vi "FFT(SubVI).vi"(0 "Data in":dbl[](array[numeric]), 1 "Window":u16, 2 "FFT size":i32, 3 "Sampling freq":dbl, 4 "Nyqvist Zone":enum32{"Zone 1", "Zone 2"}(radio)) -> (5 "Freq axis":dbl[](array[numeric]), 6 "FFT":dbl[](array[numeric]), 7 "DC Element":dbl)   [LabVIEW 2013]
uses:
  <vilib>/Analysis/4window.llb/Blackman Window (DBL).vi
  <vilib>/Analysis/4window.llb/Blackman-Harris Window (DBL).vi
  <vilib>/Analysis/4window.llb/Hamming Window (DBL).vi
  <vilib>/Analysis/4window.llb/Hanning Window (DBL).vi
  <vilib>/Analysis/2dsp.llb/Real FFT.vi
  <vilib>/Analysis/4window.llb/AllCosWindow (DBL).vi
  <vilib>/Analysis/NI_AALPro.lvlib
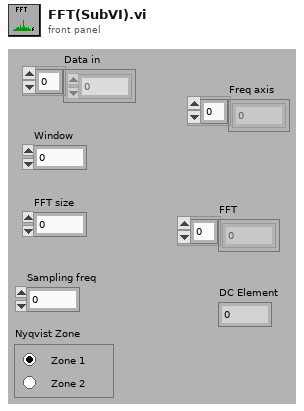
[diagram p1: front panel]
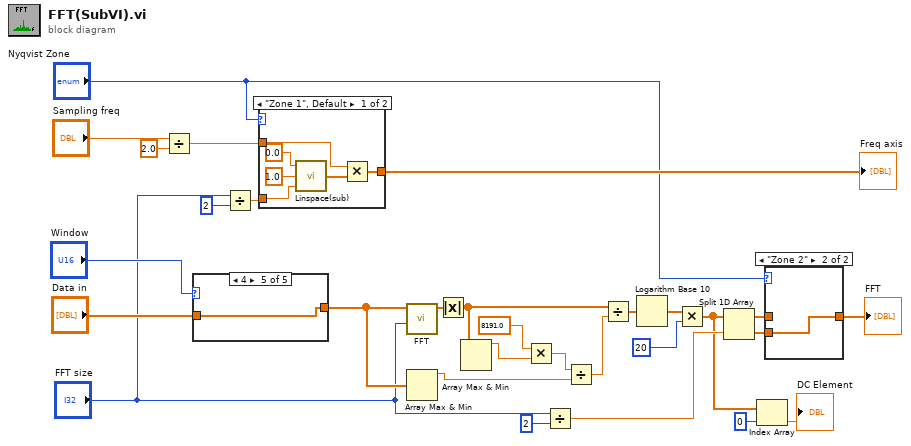
[diagram p0: block diagram]
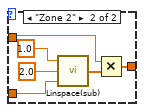
[diagram p3: hidden frame]
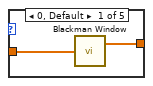
[diagram p4: hidden frame]
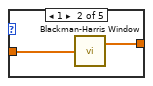
[diagram p5: hidden frame]
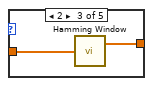
[diagram p6: hidden frame]
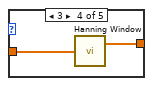
[diagram p7: hidden frame]
diagram:
  n1 = Divide(x="Sampling freq", y=2.0) -> (x/y=w17:dbl)
  n2 = case shown="4" "Window" {
    tunnel: [w31 w33 w35 w37 w38] -> w16
    tunnel: "Data in" -> [w30 w32 w34 w36 w38]
    frame 0, Default {
      n3 = call-poly <vilib>:"Blackman Window.vi"("X"=w30) -> ("Windowed X"=w31:dbl[])  [unwired: 1 out]
    }
    frame 1 {
      n4 = call-poly <vilib>:"Blackman-Harris Window.vi"("X"=w32) -> ("Windowed X"=w33:dbl[])  [unwired: 1 out]
    }
    frame 2 {
      n5 = call-poly <vilib>:"Hamming Window.vi"("X"=w34) -> ("Windowed X"=w35:dbl[])  [unwired: 1 out]
    }
    frame 3 {
      n6 = call-poly <vilib>:"Hanning Window.vi"("X"=w36) -> ("Windowed X"=w37:dbl[])  [unwired: 1 out]
    }
    frame 4 {
    }
  }
  n7 = Divide(x="FFT size", y=2) -> (x/y=w21:dbl)
  n8 = case shown="\"Zone 1\", Default" "Nyqvist Zone" {
    tunnel: w17 -> [w40 w47]
    tunnel: w21 -> [w42 w49]
    tunnel: [w39 w46] -> w22
    frame "Zone 1", Default {
      n9 = call "Linspace(sub).vi"("N of Steps"=w42, "End"=1.0 ("x"), "Start"=0.0 ("x")) -> ("Array"=w41:dbl[])
      n10 = Multiply(x=w40, y=w41) -> (x*y=w39:dbl[])
    }
    frame "Zone 2" {
      n11 = call "Linspace(sub).vi"("N of Steps"=w49, "End"=2.0 ("x"), "Start"=1.0 ("x")) -> ("Array"=w48:dbl[])
      n12 = Multiply(x=w47, y=w48) -> (x*y=w46:dbl[])
    }
  }
  "Freq axis" <- w22
  n13 = call-poly <vilib>:"FFT.vi"("FFT size"="FFT size", "X"=w16) -> ("FFT {X}"=w25:cdb[])  [unwired: 8 in, 1 out]
  n14 = Array Max & Min(array=w16) -> (max value=w14:dbl)  [unwired: 3 out]
  n15 = Absolute Value(x=w25) -> (abs(x)=w23:dbl[])
  n16 = Array Max & Min(array=w23) -> (max value=w13:dbl)  [unwired: 3 out]
  n17 = Multiply(x=8191.0, y=w13) -> (x*y=w11:dbl)
  n18 = Divide(x="FFT size", y=2) -> (x/y=w6:dbl)
  n19 = Divide(x=w11, y=w14) -> (x/y=w15:dbl)
  n20 = Divide(x=w23, y=w15) -> (x/y=w27:dbl[])
  n21 = Logarithm Base 10(1:w27) -> (0:w28:dbl[])
  n22 = Multiply(x=w28, y=20) -> (x*y=w3:dbl[])
  n23 = Split 1D Array(array=w3, index=w6) -> (first subarray=w10:dbl[], second subarray=w9:dbl[])
  n24 = Index Array(array=w3, index=0) -> (element=→"DC Element":dbl)
  n25 = case shown="\"Zone 2\"" "Nyqvist Zone" {
    tunnel: w10 -> [w51 _]
    tunnel: w9 -> [_ w52]
    tunnel: [w51 w52] -> w5
    frame "Zone 1", Default {
    }
    frame "Zone 2" {
    }
  }
  "FFT" <- w5
